vi "CloseAllVIs.vi"   [LabVIEW 2011]
doc: "This VI will close all VI's in memory."
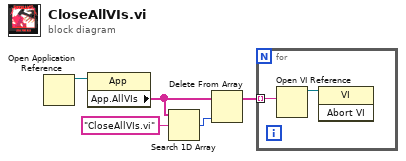
[diagram p0: block diagram]
diagram:
  n1 = Open Application Reference() -> (3:w5:refnum<vi>)  [unwired: 4 in, 1 out]
  n2 = property class="App"(reference=w5) -> ("App.AllVIs"=w3:string[])  [unwired: 1 in, 2 out]
  n3 = Search 1D Array(1D array=w3, element="CloseAllVIs.vi") -> (index of element=w1:i32)  [unwired: 1 in]
  n4 = Delete From Array(array=w3, index=w1) -> (array with subset deleted=w2:string[])  [unwired: 1 in, 1 out]
  n5 = for {
    tunnel: w2 -> [w6] mode=indexing
    n6 = Open VI Reference(vi path=w6) -> (vi reference=w7:refnum<vi>)  [unwired: 5 in, 1 out]
    n7 = invoke class="VI" method="Abort VI"(reference=w7) -> ()  [unwired: 2 in, 3 out]
  }
